vi "Read Hardware Status.vi"(8 "Error In":errorcluster, 11 "KIT-QVA in":refnum<class "KIT-QVA.lvclass">) -> (0 "Error Out":errorcluster, 3 "KIT-QVA out":refnum<class "KIT-QVA.lvclass">)   [LabVIEW 2014, in "KIT-QVA.lvlib" / "KIT-QVA.lvclass"]
doc: "Read hardware status and publish."
uses:
  KIT-QVA.lvclass
  KIT-QVA.lvclass/KIT-QVA.ctl
  instr.lib/KIT-QV/KIT QV.lvlib
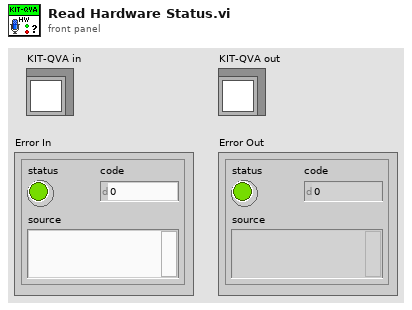
[diagram p1: front panel]
types:
  T1 = cluster{"Q1+":bool, "Q1-":bool, "Q2+":bool, "Q2-":bool, "Mute":bool, "STest-Bit":bool, "QD1":bool, "QD2":bool}
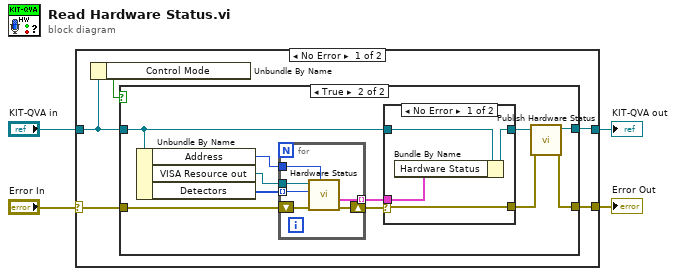
[diagram p0: block diagram]
diagram:
  n1 = case shown="No Error" "Error In" {
    selector: "Error In" -> [w9 w36]
    tunnel: [w7 w36] -> w3
    tunnel: [w8 w35] -> w1
    tunnel: "KIT-QVA in" -> [w6 w35]
    frame No Error {
      n2 = Unbundle By Name(w6) -> ("Control Mode"=w5:bool)
      n3 = case shown="True" w5 {
        tunnel: w6 -> [w11 w22]
        tunnel: w9 -> [w10 w21]
        tunnel: [w11 w14] -> w8
        tunnel: [w10 w12] -> w7
        frame False {
        }
        frame True {
          n4 = Unbundle By Name(w22) -> ("Address"=w18:u16, "VISA Resource out"=w19:refnum<visa-resource-name>, "Detectors"=w16:u8[])
          n5 = for {
            tunnel: w19 -> [w24]
            tunnel: w18 -> [w23]
            tunnel: [w26] -> w17 mode=indexing
            shift-right: [w27] -> w20
            shift-left: w21 -> [w28]
            tunnel: w16 -> [w25] mode=indexing
            n6 = call "Hardware Status.vi"("Address"=w23, "Error In"=w28, "Detector"=w25, "VISA Resource in"=w24) -> ("Error Out"=w27:errorcluster, "Hardware Cluster"=w26:T1)  [unwired: 4 in, 2 out]
          }
          n7 = case shown="No Error" w20 {
            selector: w20 -> [w29 w33]
            tunnel: w17 -> [w32 _]
            tunnel: w22 -> [w31 w34]
            tunnel: [w30 w34] -> w15
            tunnel: [w29 w33] -> w13
            frame No Error {
              n8 = Bundle By Name(cluster=w31, "Hardware Status"=w32) -> (w30:refnum<class "KIT-QVA.lvclass">)
            }
            frame Error {
            }
          }
          n9 = call "Publish Hardware Status.vi"("Error In"=w13, "KIT-QVA in"=w15) -> ("Error Out"=w12:errorcluster, "KIT-QVA out"=w14:refnum<class "KIT-QVA.lvclass">)  [unwired: 8 in]
        }
      }
    }
    frame Error {
    }
  }
  "Error Out" <- w3
  "KIT-QVA out" <- w1
